vi "Step_Change.vi"(6 "Approx Period (s)":dbl, 7 "Second array":dbl[](array[numeric])=[2.5, 2.5, 0.0, 0.0, 0.0, 0.0], 8 "Low Threshold":dbl=0.02, 9 "High Theshold":dbl=2.46, 10 "Margin Time (s)":dbl, 11 "Input Array":dbl[](array[numeric])=[2.5, 2.5, 0.0, 0.0, 0.0, 0.0]) -> (0 "Theshold index 2":i32, 1 "Theshold index 1":i32, 2 "Second array change":dbl, 3 "Analysis Type":T1)   [LabVIEW 2010]
uses:
  Controls/Step_Change.ctl
  <vilib>/Analysis/NI_AALBase.lvlib
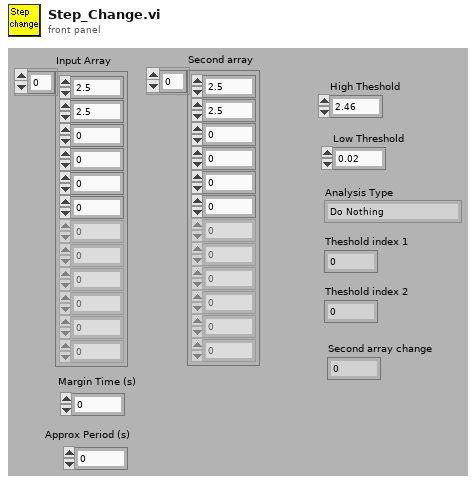
[diagram p1: front panel]
types:
  T1 = typedef "Step_Change.ctl" = enum16{"Do Nothing", "Step Up", "Step Down"}
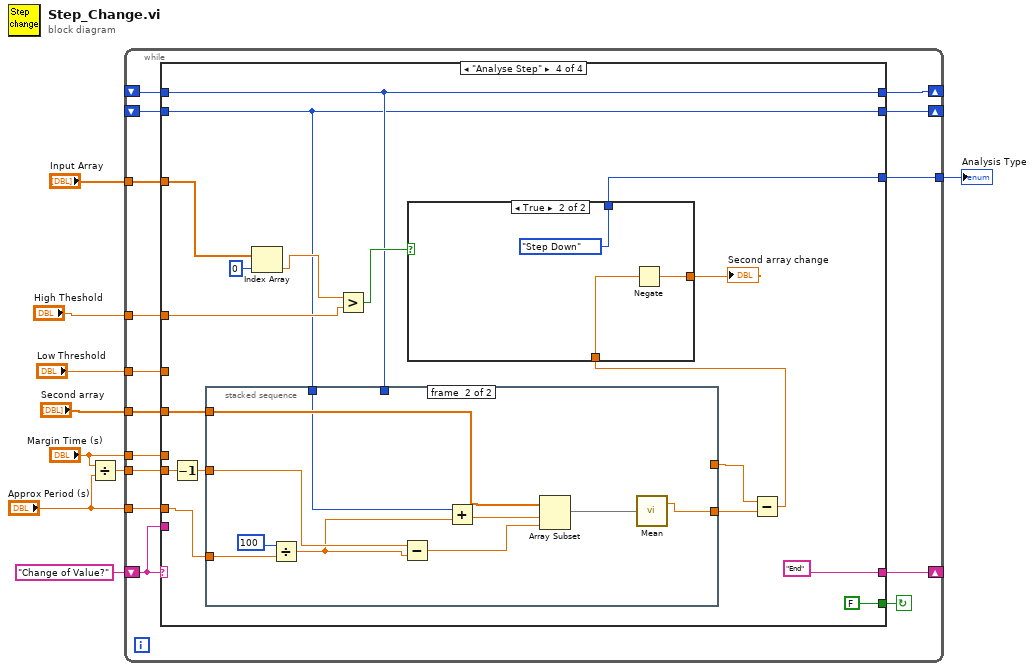
[diagram p0: block diagram]
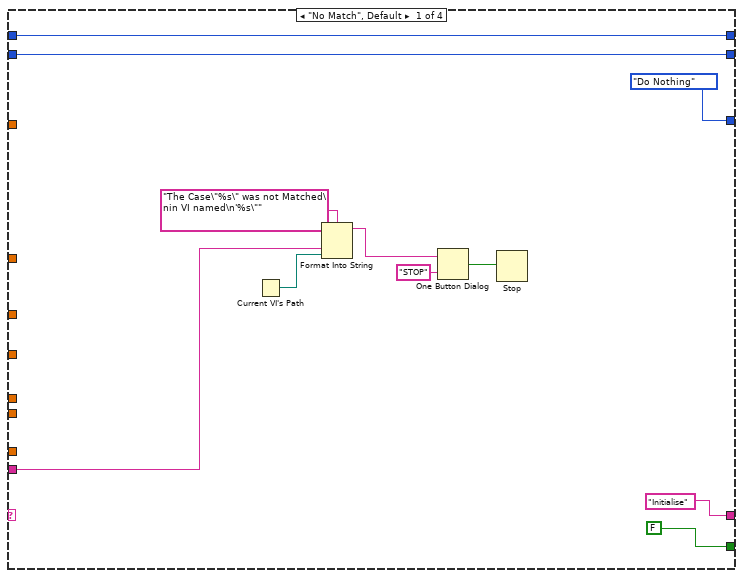
[diagram p2: hidden frame]
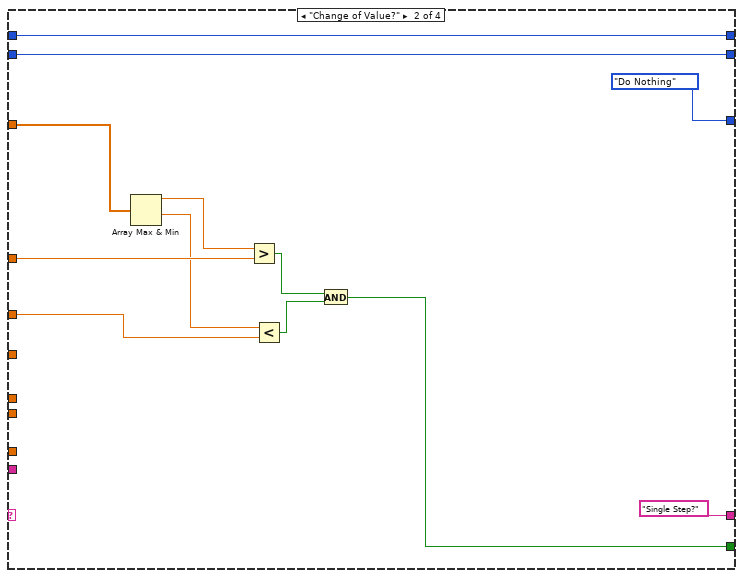
[diagram p3: hidden frame]
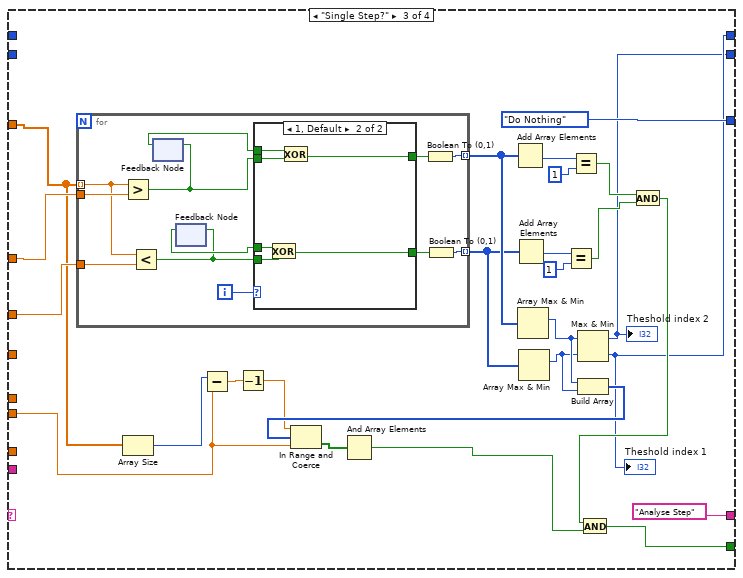
[diagram p4: hidden frame]
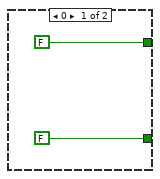
[diagram p5: hidden frame]
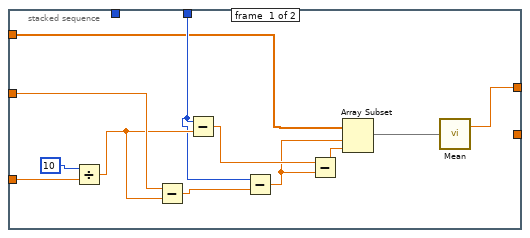
[diagram p6: hidden frame]
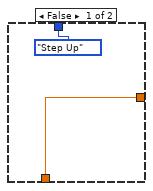
[diagram p7: hidden frame]
diagram:
  n1 = Divide(x="Margin Time (s)", y="Approx Period (s)") -> (x/y=w2:dbl)
  n2 = while {
    shift-left: "Change of Value?" -> [w22]
    shift-right: [w23] -> _
    tunnel: "Input Array" -> [w21]
    tunnel: "High Theshold" -> [w20]
    tunnel: "Low Threshold" -> [w19]
    tunnel: [w18] -> w5
    tunnel: "Margin Time (s)" -> [w17]
    tunnel: "Approx Period (s)" -> [w16]
    shift-right: [w15] -> _
    shift-left: _ -> [w13]
    shift-right: [w14] -> _
    shift-left: _ -> [w12]
    tunnel: w2 -> [w11]
    tunnel: "Second array" -> [w10]
    stop <- w24 continue-if-true
    n3 = case shown="\"Analyse Step\"" w22 {
      tunnel: [FALSE w38 w52 FALSE] -> w24
      tunnel: ["Initialise" "Single Step?" "Analyse Step" "End"] -> w23
      tunnel: w22 -> [w30 _ _ _]
      tunnel: w21 -> [_ w46 w61 w104]
      tunnel: w20 -> [_ w44 w71 w106]
      tunnel: w19 -> [_ w42 w70 _]
      tunnel: [Step_Change."Do Nothing" ("Analysis Type") Step_Change."Do Nothing" ("Analysis Type") Step_Change."Do Nothing" ("Analysis Type") w107] -> w18
      tunnel: w17 -> [_ _ _ _]
      tunnel: w16 -> [_ _ _ w103]
      tunnel: [w26 w37 w50 w101] -> w15
      tunnel: [w25 w36 w49 w99] -> w14
      tunnel: w13 -> [w26 w37 _ w101]
      tunnel: w12 -> [w25 w36 _ w99]
      tunnel: w11 -> [_ _ w48 w102]
      tunnel: w10 -> [_ _ _ w100]
      frame "No Match", Default {
        n4 = Current VI's Path() -> (path=w29:path)
        n5 = Format Into String(format string="The Case\"%s\" was not Matched\nin VI named\n'%s\"" ("Format String"), w30, w29) -> (resulting string=w33:string)  [unwired: 2 in, 1 out]
        n6 = One Button Dialog(message=w33, button name ("OK")="STOP") -> (true=w31:bool)
        n7 = Stop(stop? (T)=w31) -> ()
      }
      frame "Change of Value?" {
        n8 = Array Max & Min(array=w46) -> (max value=w45:dbl, min value=w43:dbl)  [unwired: 2 out]
        n9 = Greater?(x=w45, y=w44) -> (0:w40:bool)
        n10 = Less?(x=w43, y=w42) -> (x < y?=w41:bool)
        n11 = And(x=w40, y=w41) -> (x .and. y?=w38:bool)
      }
      frame "Single Step?" {
        n12 = for {
          tunnel: w61 -> [w80] mode=indexing
          tunnel: w71 -> [w85]
          tunnel: [w82] -> w63 mode=indexing
          tunnel: w70 -> [w79]
          tunnel: [w76] -> w62 mode=indexing
          i -> [w74]
          n13 = Greater?(x=w80, y=w85) -> (0:w84:bool)
          n14 = Less?(x=w80, y=w79) -> (x < y?=w77:bool)
          n15 = feedback-in #1(w84) -> ()
          n16 = feedback #1() -> (w81:bool)  [unwired: 1 in]
          n17 = feedback-in #2(w77) -> ()
          n18 = feedback #2() -> (w78:bool)  [unwired: 1 in]
          n19 = case shown="1, Default" w74 {
            tunnel: w84 -> [_ w93]
            tunnel: [FALSE w88] -> w83
            tunnel: w81 -> [_ w92]
            tunnel: w78 -> [_ w91]
            tunnel: w77 -> [_ w90]
            tunnel: [FALSE w89] -> w75
            frame 0 {
            }
            frame 1, Default {
              n20 = Exclusive Or(1:w90, 2:w91) -> (0:w89:bool)
              n21 = Exclusive Or(1:w93, 2:w92) -> (0:w88:bool)
            }
          }
          n22 = Boolean To (0,1)(Boolean=w83) -> (0, 1=w82:i16)
          n23 = Boolean To (0,1)(Boolean=w75) -> (0, 1=w76:i16)
        }
        n24 = Array Size(array=w61) -> (size(s)=w60:i32)
        n25 = Subtract(x=w60, y=w48) -> (x-y=w59:dbl)
        n26 = Decrement(x=w59) -> (x-1=w51:dbl)
        n27 = Add Array Elements(numeric array=w63) -> (sum=w69:i16)
        n28 = Add Array Elements(numeric array=w62) -> (sum=w66:i16)
        n29 = Array Max & Min(array=w63) -> (max index (indices)=w58:i32)  [unwired: 3 out]
        n30 = Array Max & Min(array=w62) -> (max index (indices)=w57:i32)  [unwired: 3 out]
        n31 = Equal?(x=w66, y=i16 1) -> (x = y?=w65:bool)
        n32 = Equal?(x=w69, y=i16 1) -> (x = y?=w64:bool)
        n33 = Max & Min(x=w58, y=w57) -> (max(x,y)=w49:i32, min(x,y)=w50:i32)
        "Theshold index 1" <- w50
        "Theshold index 2" <- w49
        n34 = Build Array(w58, w57) -> (w56:i32[])
        n35 = In Range and Coerce(upper limit=w51, x=w56, lower limit=w48) -> (In Range?=w55:bool[])  [unwired: 1 out]
        n36 = And Array Elements(Boolean array=w55) -> (logical AND=w53:bool)
        n37 = And(x=w64, y=w65) -> (x .and. y?=w54:bool)
        n38 = And(x=w54, y=w53) -> (x .and. y?=w52:bool)
      }
      frame "Analyse Step" {
        n39 = Decrement(x=w102) -> (x-1=w96:dbl)
        n40 = stacked-sequence {
          tunnel: w103 -> [w122 w132]
          tunnel: w96 -> [w121 w127]
          tunnel: w101 -> [w119 _]
          tunnel: w100 -> [w114 w131]
          tunnel: [w112 _] -> w98
          tunnel: w99 -> [_ w129]
          tunnel: [_ w124] -> w97
          frame #0 {
            n41 = Divide(x=10, y=w122) -> (x/y=w120:dbl)
            n42 = Subtract(x=w121, y=w120) -> (x-y=w118:dbl)
            n43 = Subtract(x=w119, y=w120) -> (x-y=w117:dbl)
            n44 = Subtract(x=w119, y=w118) -> (x-y=w116:dbl)
            n45 = Subtract(x=w117, y=w116) -> (x-y=w115:dbl)
            n46 = Array Subset(array=w114, index=w116, length=w115) -> (w113:dbl[])
            n47 = call <vilib>:"Mean.vi"("X"=w113) -> ("mean"=w112:dbl)  [unwired: 1 out]
          }
          frame #1 {
            n48 = Divide(x=100, y=w132) -> (x/y=w126:dbl)
            n49 = Subtract(x=w127, y=w126) -> (x-y=w125:dbl)
            n50 = Add(x=w129, y=w126) -> (x+y=w128:dbl)
            n51 = Array Subset(array=w131, index=w128, length=w125) -> (w130:dbl[])
            n52 = call <vilib>:"Mean.vi"("X"=w130) -> ("mean"=w124:dbl)  [unwired: 1 out]
          }
        }
        n53 = Index Array(array=w104, index=0) -> (element=w109:dbl)
        n54 = Greater?(x=w109, y=w106) -> (0:w108:bool)
        n55 = Subtract(x=w98, y=w97) -> (x-y=w94:dbl)
        n56 = case shown="True" w108 {
          tunnel: [Step_Change."Step Up" ("Analysis Type") Step_Change."Step Down" ("Analysis Type")] -> w107
          tunnel: [w134 w136] -> w95
          tunnel: w94 -> [w134 w137]
          frame False {
          }
          frame True {
            n57 = Negate(x=w137) -> (-x=w136:dbl)
          }
        }
        "Second array change" <- w95
      }
    }
  }
  "Analysis Type" <- w5
